vi "crazy crap.vi"(7 "error in":errorcluster) -> (27 "error out":errorcluster)   [LabVIEW 2012]
panel:
  out "Image Out":T1(plugin-control)
  out "Histogram Graph":u32[][](graph)
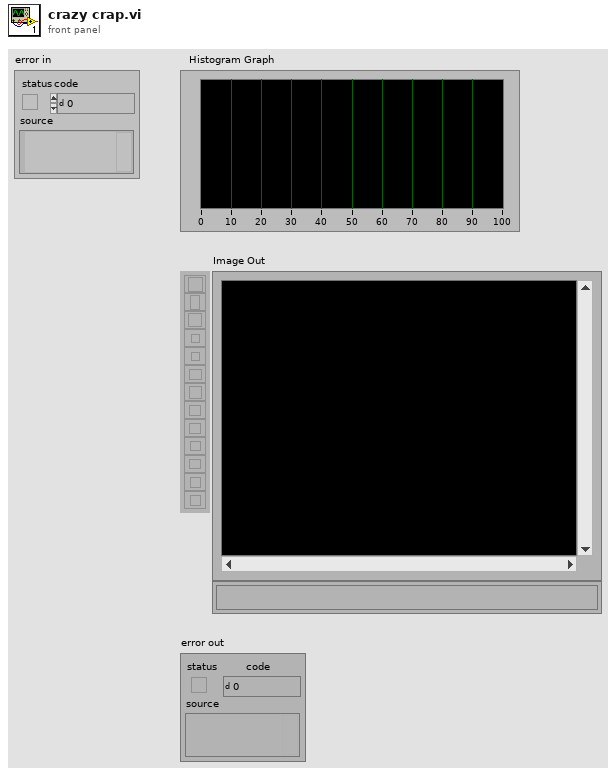
[diagram p1: front panel]
types:
  T1 = typedef "IMAQ Image.ctl" = refnum<image>
  T2 = cluster{"Global Rectangle":i32[], "Contours":cluster{"ID":enum32{"External", "Internal"}, "Type":u32, "Coordinates":i32[]}[]}
  T3 = typedef "Image Type" = u32
  T4 = cluster{"Minimal Value":sgl, "Maximal Value":sgl, "Mean Value":sgl, "Standard  Variation":sgl, "Area (pixels)":i32}
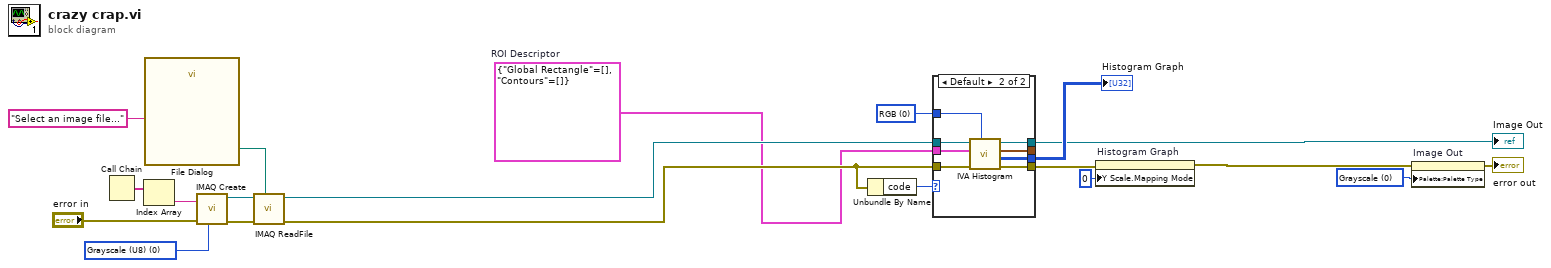
[diagram p0: block diagram]
diagram:
  w2 = u32 0 items=["Grayscale", "Binary", "Gradient", "Rainbow", "Temperature", "User Defined"] ("Palette")
  w8 = u16 0 items=["RGB", "HSL", "HSV", "HSI"] ("Color Mode")
  w6 = T2 {"Global Rectangle"=[], "Contours"=[]}  # ROI Descriptor
  w12 = T3 0 items=["Grayscale (U8)", "Grayscale (I16)", "Grayscale (SGL)", "Complex (CSG)", "RGB (U32)", "HSL (U32)", "RGB (U64)", "Grayscale (U16)"] ("Image Type")
  n1 = Call Chain() -> (call chain=w16:string[])
  n2 = Index Array(array=w16) -> (element=w15:string)  [unwired: 1 in]
  n3 = call "File Dialog"("prompt"="Select an image file...") -> ("selected path"=w13:path)  [unwired: 6 in, 8 out]
  n4 = call "IMAQ Create"("Image Name"=w15, "Image Type"=w12, "error in (no error)"="error in") -> ("New Image"=w19:T1, "error out"=w18:errorcluster)  [unwired: 1 in, 1 out]
  n5 = call "IMAQ ReadFile"("File Path"=w13, "error in (no error)"=w18, "Image"=w19) -> ("error out"=w20:errorcluster, "Image Out"=w11:T1)  [unwired: 2 in, 5 out]
  n6 = Unbundle By Name(w20) -> ("code"=w4:i32)
  n7 = case shown="Default" w4 {
    tunnel: w20 -> [_ w29]
    tunnel: w11 -> [w21 w28]
    tunnel: [_ w27] -> _
    tunnel: [_ w26] -> w9
    tunnel: w8 -> [_ w25]
    tunnel: [_ w24] -> w7
    tunnel: w6 -> [_ w23]
    tunnel: [w21 w22] -> w3
    frame -1074396199, -1074396198 {
      # "Discard\nCoordinate\nSystem\nError"
    }
    frame Default {
      n8 = call <vilib>:"IVA Histogram.vi"("Color Mode"=w25, "error in (no error)"=w29, "ROI Descriptor"=w23, "Image In"=w28) -> ("error out"=w26:errorcluster, "Histograms"=w24:u32[][], "Statistics"=w27:T4, "Image Out"=w22:T1)  [unwired: 4 out]
    }
  }
  "Histogram Graph" <- w7
  "Image Out" <- w3
  n9 = property on="Histogram Graph" class="WFGraph (strict)"(error in=w9, "Y Scale.Mapping Mode"=u8 0) -> (error out=w5:errorcluster)  [unwired: 1 in, 1 out]
  n10 = property on="Image Out" class="ImageControl"(error in=w5, "Palette:Palette Type"=w2) -> (error out=→"error out":errorcluster)  [unwired: 1 in, 1 out]
